vi "Puzzle 4-2.vi"() -> ()   [LabVIEW 2022 SP3]
panel:
  out "sum":i32
  out "Array":i32[](array[numeric])
  in  "delimited string":string
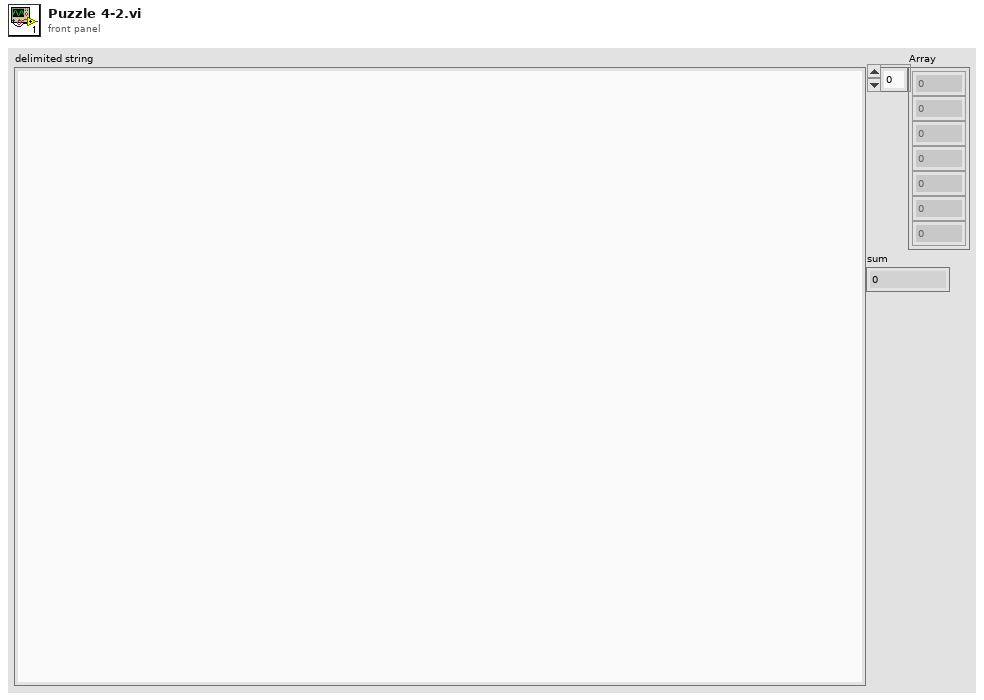
[diagram p1: front panel]
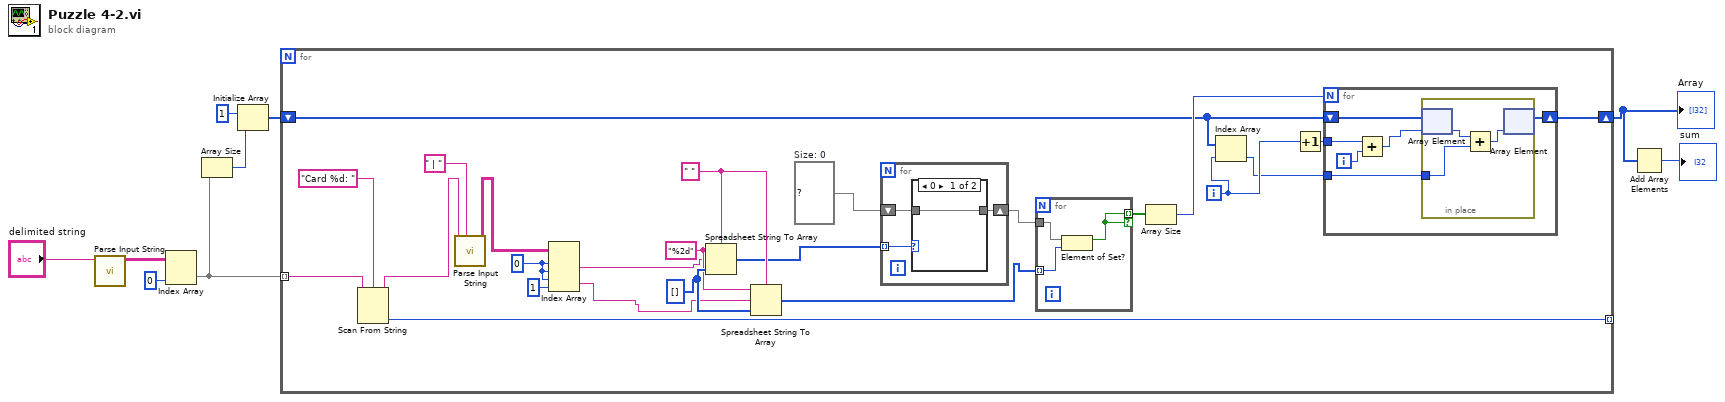
[diagram p0: block diagram]
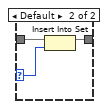
[diagram p2: hidden frame]
diagram:
  n1 = call "Parse Input String.vi"("delimited string"="delimited string") -> ("parsed string"=w8:string[][])  [unwired: 10 in]
  n2 = Index Array(array=w8, index (col)=0 ("disabled index (col)")) -> (element=w4:string[])  [unwired: 1 in]
  n3 = Array Size(array=w4) -> (size(s)=w5:i32)
  n4 = Initialize Array(1 ("element"), w5) -> (w3:i32[])
  n5 = for {
    tunnel: w4 -> [w33] mode=indexing
    tunnel: [w31] -> _ mode=indexing
    shift-right: [w15] -> w2
    shift-left: w3 -> [w12]
    i -> [w11]
    w19 = set{i32} {}  # Size: 0
    w26 = i32[] [] ("array type (2D Dbl)")
    w25 = "%2d" ("format string")
    w27 = " " ("delimiter (Tab)")
    w24 = 0 ("disabled index (col)")
    n6 = Scan From String(format string="Card %d: " ("delimiter (Tab)"), input string=w33) -> (remaining string=w30:string, output 1=w31:i32)  [unwired: 3 in, 2 out]
    n7 = call "Parse Input String.vi"("delimiter (Tab)"=" | ", "delimited string"=w30) -> ("parsed string"=w28:string[][])  [unwired: 9 in]
    n8 = Index Array(array=w28, index (row) #1=w24, index (col) #1=w24, index (row) #2=w24, index (col) #2=1 ("disabled index (col)")) -> (element #1=w22:string, element #2=w21:string)
    n9 = Spreadsheet String To Array(delimiter (Tab)=w27, format string=w25, spreadsheet string=w22, array type (2D Dbl)=w26) -> (array=w20:i32[])
    n10 = Spreadsheet String To Array(delimiter (Tab)=w27, format string=w25, spreadsheet string=w21, array type (2D Dbl)=w26) -> (array=w18:i32[])
    n11 = for {
      tunnel: w20 -> [w48] mode=indexing
      shift-right: [w47] -> w17
      shift-left: w19 -> [w46]
      n12 = case shown="0" w48 {
        selector: w48 -> [_ w52]
        tunnel: [w49 w51] -> w47
        tunnel: w46 -> [w49 w50]
        frame 0 {
        }
        frame Default {
          n13 = Insert Into Set(10:w52, 11:w50) -> (3:w51:set{i32})  [unwired: 1 out]
        }
      }
    }
    n14 = for {
      tunnel: w18 -> [w44] mode=indexing
      tunnel: w17 -> [w45]
      tunnel: [w43] -> w16 mode=indexing if=w43
      n15 = Element of Set?(10:w44, 11:w45) -> (3:w43:bool)
    }
    n16 = Array Size(array=w16) -> (size(s)=w14:i32)
    n17 = Index Array(array=w12, index=w11) -> (element=w10:i32)
    n18 = Increment(x=w11) -> (x+1=w13:i32)
    n19 = for {
      N: w14 -> [_]
      shift-right: [w35] -> w15
      shift-left: w12 -> [w39]
      tunnel: w13 -> [w37]
      tunnel: w10 -> [w34]
      i -> [w38]
      n20 = Add(x=w37, y=w38) -> (x+y=w36:i32)
      n21 = in-place {
        in-place-border: w34 -> [w40]
        n22 = in-place-array #1(w39, w36) -> (w42:i32)
        n23 = Add(x=w42, y=w40) -> (x+y=w41:i32)
        n24 = in-place-array #1(w41) -> (w35:i32[])  [unwired: 1 out]
      }
    }
  }
  "Array" <- w2
  n25 = Add Array Elements(numeric array=w2) -> (sum=→"sum":i32)
